vi "dateBreakdown.vi"(11 "seconds since 1Jan1904":timestamp=timestamp(-126147600 s since 1904-01-01) format="%<%H:%M:%S %Z\n%Y/%m/%d>T") -> (1 "dateElementsArray":cluster{"chName":string, "chValue":string}[](array[cluster]))   [LabVIEW 2021]
uses:
  <vilib>/Utility/miscctls.llb/LVDateTimeRec.ctl
panel:
  out "Excel:Days:Since1900-1-1":dbl format="%#.6g"
  out "Date:Plottable":string
  out "Month:Name":string
  out "Day:Of:Year":string
  out "Date:Sortable":string
  out "Seconds:Since:Midnight":dbl
  out "Day:Of:Month":string
  out "Month:Num":string
  out "Day:Of:Week":string
  out "Day:Name":string
  out "Year":string
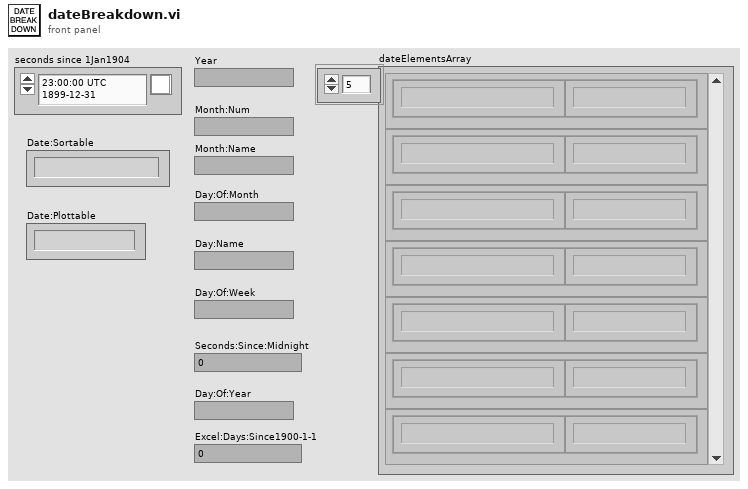
[diagram p1: front panel]
types:
  T1 = typedef "LVDateTimeRec.ctl" = cluster{"fractional second":dbl, "second":i32, "minute":i32, "hour":i32, "day of month":i32, "month":i32, "year":i32, "day of week":i32, "day of year":i32, "DST":i32}
  T2 = cluster{"Label.Text":string, "date/time string":string}
  T3 = cluster{"Label.Text":string, "date/time string":string}[]
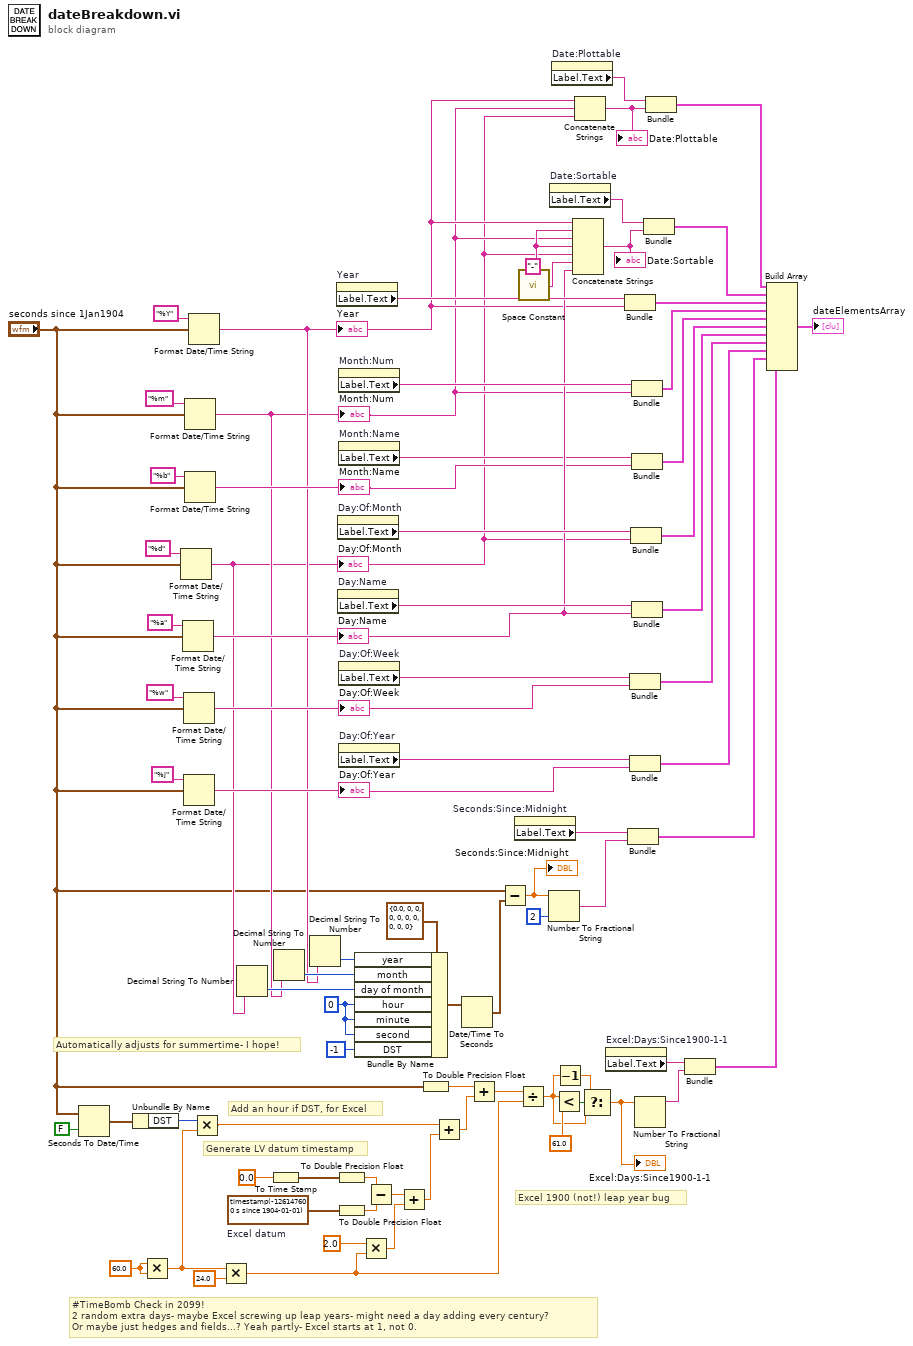
[diagram p0: block diagram]
diagram:
  w10 = 60.0 ("value")
  w26 = timestamp(-126147600 s since 1904-01-01)  # Excel datum
  w43 = "-" ("string")
  w78 = 0 ("hour")
  # "Add an hour if DST, for Excel"
  # "Excel 1900 (not!) leap year bug"
  # "#TimeBomb Check in 2099!\n2 random extra days- maybe Excel screwing up leap years- might need a day adding every century?\nOr maybe just hedges and fields...? Yeah partly- Excel starts at 1, not 0."
  # "Generate LV datum timestamp"
  # "Automatically adjusts for summertime- I hope!"
  n1 = Seconds To Date/Time(time stamp (now)="seconds since 1Jan1904", to UTC (F)=FALSE) -> (date time rec=w12:T1)
  n2 = Unbundle By Name(w12) -> ("DST"=w9:i32)
  n3 = Multiply(x=w10, y=w10) -> (x*y=w8:dbl)
  n4 = Format Date/Time String(time format string (%c)="%d", seconds (now)="seconds since 1Jan1904") -> (date/time string=w31:string)  [unwired: 1 in]
  "Day:Of:Month" <- w31
  n5 = Format Date/Time String(time format string (%c)="%a", seconds (now)="seconds since 1Jan1904") -> (date/time string=w42:string)  [unwired: 1 in]
  "Day:Name" <- w42
  n6 = Format Date/Time String(time format string (%c)="%w", seconds (now)="seconds since 1Jan1904") -> (date/time string=w50:string)  [unwired: 1 in]
  "Day:Of:Week" <- w50
  n7 = Format Date/Time String(time format string (%c)="%j", seconds (now)="seconds since 1Jan1904") -> (date/time string=w48:string)  [unwired: 1 in]
  "Day:Of:Year" <- w48
  n8 = Format Date/Time String(time format string (%c)="%m", seconds (now)="seconds since 1Jan1904") -> (date/time string=w32:string)  [unwired: 1 in]
  "Month:Num" <- w32
  n9 = Format Date/Time String(time format string (%c)="%b", seconds (now)="seconds since 1Jan1904") -> (date/time string=w40:string)  [unwired: 1 in]
  "Month:Name" <- w40
  n10 = Format Date/Time String(time format string (%c)="%Y", seconds (now)="seconds since 1Jan1904") -> (date/time string=w33:string)  [unwired: 1 in]
  "Year" <- w33
  n11 = Multiply(x=w9, y=w8) -> (x*y=w6:dbl)
  n12 = Multiply(x=w8, y=24.0 ("value")) -> (x*y=w16:dbl)
  n13 = Decimal String To Number(string=w31) -> (number=w76:i32)  [unwired: 2 in, 1 out]
  n14 = To Time Stamp(1:0.0) -> (0:w25:timestamp)
  n15 = Decimal String To Number(string=w32) -> (number=w75:i32)  [unwired: 2 in, 1 out]
  n16 = Decimal String To Number(string=w33) -> (number=w74:i32)  [unwired: 2 in, 1 out]
  n17 = property on="Year" class="Str"() -> ("Label.Text"=w55:string)  [unwired: 2 in, 2 out]
  n18 = To Double Precision Float(number=w25) -> (double precision float=w22:dbl)
  n19 = To Double Precision Float(number=w26) -> (double precision float=w21:dbl)
  n20 = property on="Day:Of:Month" class="Str"() -> ("Label.Text"=w53:string)  [unwired: 2 in, 2 out]
  n21 = property on="Day:Name" class="Str"() -> ("Label.Text"=w52:string)  [unwired: 2 in, 2 out]
  n22 = property on="Month:Num" class="Str"() -> ("Label.Text"=w54:string)  [unwired: 2 in, 2 out]
  n23 = property on="Month:Name" class="Str"() -> ("Label.Text"=w39:string)  [unwired: 2 in, 2 out]
  n24 = property on="Day:Of:Week" class="Str"() -> ("Label.Text"=w51:string)  [unwired: 2 in, 2 out]
  n25 = property on="Day:Of:Year" class="Str"() -> ("Label.Text"=w49:string)  [unwired: 2 in, 2 out]
  n26 = Bundle By Name(cluster=T1 {"fractional second"=0.0, "second"=0, "minute"=0, "hour"=0, "day of month"=0, "month"=0, "year"=0, "day of week"=0, "day of year"=0, "DST"=0} ("date time rec"), "year"=w74, "month"=w75, "day of month"=w76, "hour"=w78, "minute"=w78, "second"=w78, "DST"=-1) -> (w72:T1)
  n27 = Multiply(x=2.0, y=w16) -> (x*y=w17:dbl)
  n28 = Subtract(x=w22, y=w21) -> (x-y=w20:dbl)
  n29 = Add(x=w20, y=w17) -> (x+y=w19:dbl)
  n30 = To Double Precision Float(number="seconds since 1Jan1904") -> (double precision float=w23:dbl)
  n31 = Add(x=w6, y=w19) -> (x+y=w7:dbl)
  n32 = Date/Time To Seconds(2:w72) -> (0:w77:timestamp)  [unwired: 1 in]
  n33 = Add(x=w23, y=w7) -> (x+y=w24:dbl)
  n34 = Subtract(x="seconds since 1Jan1904", y=w77) -> (x-y=w66:dbl)
  "Seconds:Since:Midnight" <- w66
  n35 = property on="Seconds:Since:Midnight" class="DigNum (strict)"() -> ("Label.Text"=w47:string)  [unwired: 2 in, 2 out]
  n36 = Divide(x=w24, y=w16) -> (x/y=w3:dbl)
  n37 = call <vilib>:"Space Constant.vi"() -> ("String"=w41:string)
  n38 = Number To Fractional String(number=w66, precision (6)=i16 2) -> (F-format string=w46:string)  [unwired: 2 in]
  n39 = property on="Date:Sortable" class="Str"() -> ("Label.Text"=w45:string)  [unwired: 2 in, 2 out]
  n40 = property on="Date:Plottable" class="Str"() -> ("Label.Text"=w34:string)  [unwired: 2 in, 2 out]
  n41 = Less?(x=w3, y=61.0) -> (x < y?=w1:bool)
  n42 = Decrement(x=w3) -> (x-1=w4:dbl)
  n43 = Concatenate Strings(w33, w43, w32, w43, w31, w41, w42) -> (w44:string)
  "Date:Sortable" <- w44
  n44 = Concatenate Strings(w33, w32, w31) -> (w35:string)
  "Date:Plottable" <- w35
  n45 = Select(t=w4, s=w1, f=w3) -> (s? t:f=w2:dbl)
  "Excel:Days:Since1900-1-1" <- w2
  n46 = property on="Excel:Days:Since1900-1-1" class="DigNum (strict)"() -> ("Label.Text"=w29:string)  [unwired: 2 in, 2 out]
  n47 = Bundle("Label.Text"=w55, "date/time string"=w33) -> (w64:T2)  [unwired: 1 in]
  n48 = Bundle("Label.Text"=w47, w46) -> (w57:cluster{"Label.Text":string, string})  [unwired: 1 in]
  n49 = Bundle("Label.Text"=w51, "date/time string"=w50) -> (w61:T2)  [unwired: 1 in]
  n50 = Bundle("Label.Text"=w49, "date/time string"=w48) -> (w56:T2)  [unwired: 1 in]
  n51 = Bundle("Label.Text"=w53, "date/time string"=w31) -> (w37:T2)  [unwired: 1 in]
  n52 = Bundle("Label.Text"=w54, "date/time string"=w32) -> (w63:T2)  [unwired: 1 in]
  n53 = Bundle("Label.Text"=w39, "date/time string"=w40) -> (w36:T2)  [unwired: 1 in]
  n54 = Bundle("Label.Text"=w52, "date/time string"=w42) -> (w62:T2)  [unwired: 1 in]
  n55 = Number To Fractional String(number=w2) -> (F-format string=w14:string)  [unwired: 3 in]
  n56 = Bundle("Label.Text"=w45, w44) -> (w59:cluster{"Label.Text":string, string})  [unwired: 1 in]
  n57 = Bundle("Label.Text"=w34, w35) -> (w30:cluster{"Label.Text":string, string})  [unwired: 1 in]
  n58 = Bundle("Label.Text"=w29, w14) -> (w15:cluster{"Label.Text":string, string})  [unwired: 1 in]
  n59 = Build Array(w30, w59, w64, w63, w36, w37, w62, w61, w56, w57, w15) -> (→"dateElementsArray":T3)
